vi "XY Galvo Generator.vi"(0 "Exposure /ms":dbl, 1 "FOV max / V":dbl, 2 "Samples per ms":dbl, 3 "Relax /ms":dbl, 4 "FOV min/ V":dbl, 7 "Delay /ms":dbl) -> (5 "Signal":dbl[](array[numeric]))   [LabVIEW 2015]
uses:
  <vilib>/Analysis/1siggen.llb/Ramp Pattern by Samples.vi
  <vilib>/Analysis/NI_AALBase.lvlib
panel:
  out "Underscan":dbl[](graph)
  in  "Underscan /ms":dbl
  out "XY Galvo":dbl[](graph)
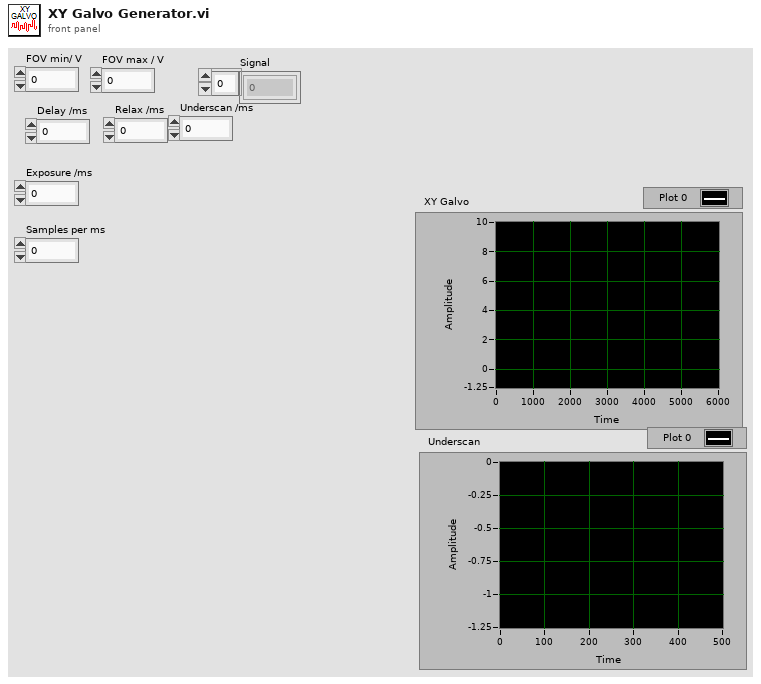
[diagram p1: front panel]
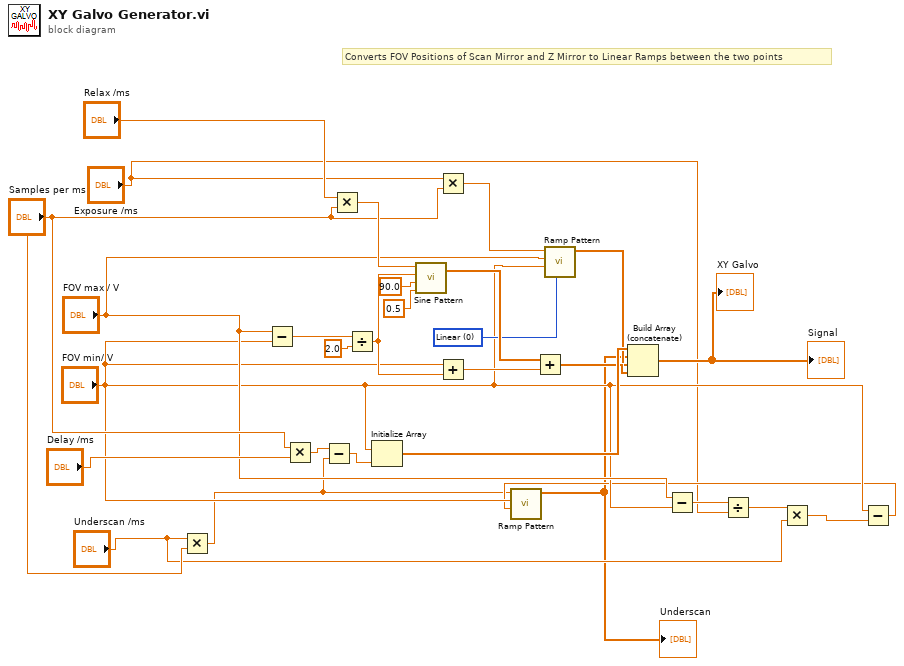
[diagram p0: block diagram]
diagram:
  w19 = u16 0 items=["Linear", "Logarithmic"] ("type")
  # "Converts FOV Positions of Scan Mirror and Z Mirror to Linear Ramps between the two points"
  n1 = Multiply(x="Underscan /ms", y="Samples per ms") -> (x*y=w5:dbl)
  n2 = Subtract(x="FOV max / V", y="FOV min/ V") -> (x-y=w26:dbl)
  n3 = Multiply(x="Samples per ms", y="Delay /ms") -> (x*y=w6:dbl)
  n4 = Subtract(x=w6, y=w5) -> (x-y=w4:dbl)
  n5 = Multiply(x="Relax /ms", y="Samples per ms") -> (x*y=w24:dbl)
  n6 = Divide(x=w26, y=2.0 ("phase(degrees)")) -> (x/y=w29:dbl)
  n7 = Initialize Array("FOV min/ V", w4) -> (w16:dbl[])
  n8 = call <vilib>:"Sine Pattern.vi"("cycles"=0.5, "phase(degrees)"=90.0, "amplitude"=w29, "samples"=w24) -> ("Sinusoidal Pattern"=w20:dbl[])  [unwired: 1 out]
  n9 = Multiply(x="Exposure /ms", y="Samples per ms") -> (x*y=w22:dbl)
  n10 = Add(x="FOV min/ V", y=w29) -> (x+y=w28:dbl)
  n11 = Add(x=w20, y=w28) -> (x+y=w3:dbl[])
  n12 = call-poly <vilib>:"Ramp Pattern.vi"("type"=w19, "start"="FOV min/ V", "end"="FOV max / V", "samples"=w22) -> ("Ramp Pattern"=w2:dbl[])  [unwired: 6 in, 1 out]
  n13 = Subtract(x="FOV max / V", y="FOV min/ V") -> (x-y=w8:dbl)
  n14 = Divide(x=w8, y="Exposure /ms") -> (x/y=w13:dbl)
  n15 = Multiply(x=w13, y="Underscan /ms") -> (x*y=w11:dbl)
  n16 = Subtract(x="FOV min/ V", y=w11) -> (x-y=w10:dbl)
  n17 = call-poly <vilib>:"Ramp Pattern.vi"("start"=w10, "end"="FOV min/ V", "samples"=w5) -> ("Ramp Pattern"=w1:dbl[])  [unwired: 7 in, 1 out]
  "Underscan" <- w1
  n18 = Build Array (concatenate)(w16, w1, w2, w3) -> (→"Signal" →"XY Galvo":dbl[])
